vi "send handshake response.vi"(9 "supported protocols":string[](array[string]), 10 "return sec key":string, 11 "TCP Network Connection in":refnum<k5>) -> (0 "error out":errorcluster)   [LabVIEW 2016, in "websocket standalone server.lvclass"]
uses:
  websocket standalone server.lvclass
  HTTP server/http response.ctl
  HTTP server/http response packet type.ctl
  HTTP headers/http header data.ctl
  HTTP server/Basic HTTP server.lvclass
  HTTP headers/http headers.lvlib
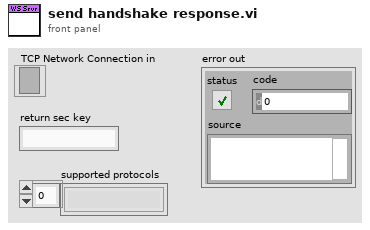
[diagram p1: front panel]
types:
  T1 = typedef "Basic HTTP server.lvclass/http response packet type.ctl" = enum16{"full response", "header only", "data only", "last data"}
  T2 = typedef "Basic HTTP server.lvclass/http response.ctl" = cluster{"packet type":T1, "reason code":u16, "status string":string, "headers":T3, "cookies":string[], "data":string}
  T3 = typedef "http headers.lvlib/http header data.ctl" = cluster{"fields":string[], "values":string[]}
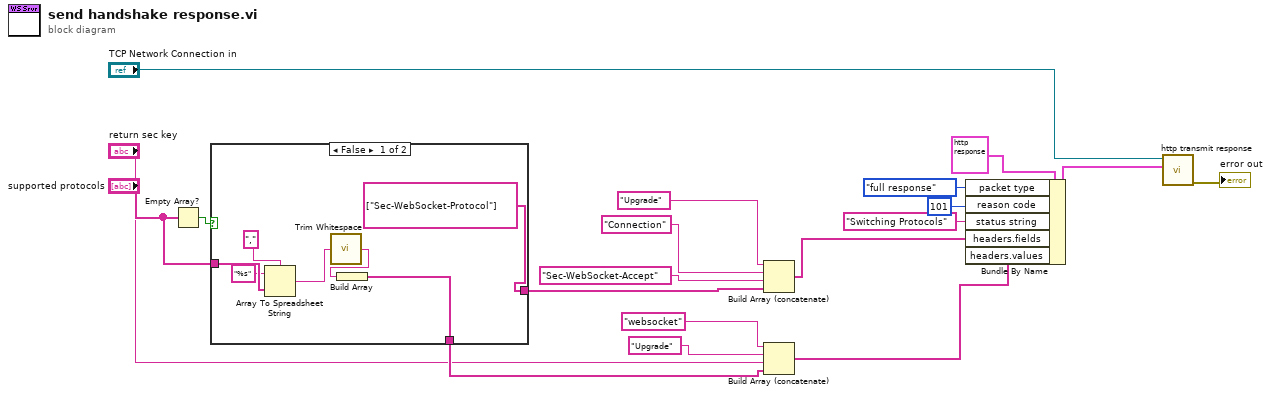
[diagram p0: block diagram]
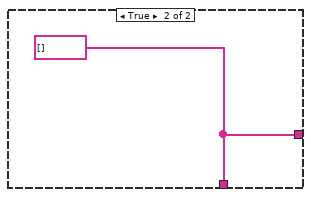
[diagram p2: hidden frame]
diagram:
  n1 = Empty Array?(array="supported protocols") -> (empty?=w16:bool)
  n2 = case shown="False" w16 {
    tunnel: [string[] ["Sec-WebSocket-Protocol"] ("appended array") w27] -> w17
    tunnel: [w24 w27] -> w18
    tunnel: "supported protocols" -> [w22 _]
    frame False {
      n3 = Array To Spreadsheet String(delimiter (Tab)=",", array=w22, 3:"%s" ("format string")) -> (spreadsheet string=w23:string)
      n4 = call <vilib>:"Trim Whitespace.vi"("string"=w23) -> ("trimmed string"=w25:string)  [unwired: 1 in]
      n5 = Build Array(w25) -> (w24:string[])
    }
    frame True {
      w27 = string[] [] ("appended array")
    }
  }
  n6 = Build Array (concatenate)("Upgrade" ("status string"), "Connection" ("status string"), "Sec-WebSocket-Accept" ("status string"), w17) -> (w9:string[])
  n7 = Build Array (concatenate)("websocket" ("status string"), "Upgrade" ("status string"), "return sec key", w18) -> (w10:string[])
  n8 = Bundle By Name(cluster=T2 {"packet type"=enum."full response", "reason code"=101, "status string"="", "headers"={"fields"=[], "values"=[]}, "cookies"=[], "data"=""} ("application request"), "packet type"=http_response_packet_type."full response", "reason code"=u16 101, "status string"="Switching Protocols", "headers.fields"=w9, "headers.values"=w10) -> (w2:T2)
  n9 = call "http transmit response.vi"("application request"=w2, "tcp connection"="TCP Network Connection in") -> ("error out"=→"error out":errorcluster)  [unwired: 9 in]
